vi "Special_Case_Mistake_Resolve-1.vi"(1 "[IN] Subtracks":T1(array[cluster]), 2 "[IN] Index of \nBest Subtrack":i32) -> (0 "[OUT] FALSE For Pre\nventing double save":bool)   [LabVIEW 2013]
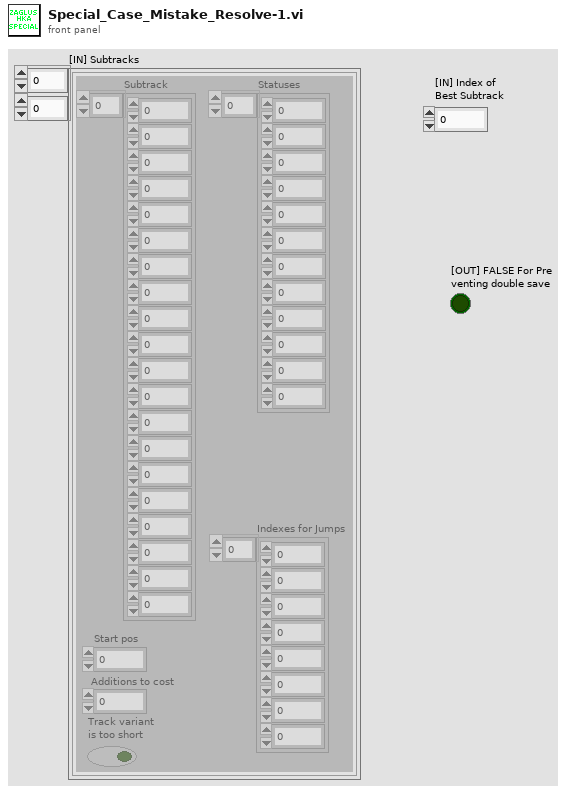
[diagram p1: front panel]
types:
  T1 = cluster{"Subtrack":dbl[], "Statuses":i16[], "Start pos":i32, "Additions to cost":i32, "Track variant \nis too short":bool, "Indexes for Jumps":i32[]}[][]
  T2 = cluster{"Subtrack":dbl[], "Statuses":i16[], "Start pos":i32, "Additions to cost":i32, "Track variant \nis too short":bool, "Indexes for Jumps":i32[]}
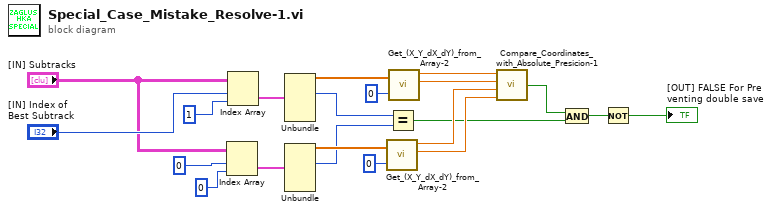
[diagram p0: block diagram]
diagram:
  n1 = Index Array(array="[IN] Subtracks", index (row)=0, index (col)=0 ("index (row)")) -> (element=w16:T2)
  n2 = Index Array(array="[IN] Subtracks", index (row)="[IN] Index of \nBest Subtrack", index (col)=1 ("disabled index (col)")) -> (element=w20:T2)
  n3 = Unbundle(w20) -> ("Subtrack"=w15:dbl[], "Start pos"=w11:i32)  [unwired: 4 out]
  n4 = Unbundle(w16) -> ("Subtrack"=w12:dbl[], "Start pos"=w10:i32)  [unwired: 4 out]
  n5 = call "Get_(X_Y_dX_dY)_from_Array-2.vi"("(X,Y,dX,dY)"=w12, "Index of Displacement"=0) -> ("X"=w7:dbl, "Y"=w6:dbl)  [unwired: 2 out]
  n6 = Equal?(x=w11, y=w10) -> (x = y?=w4:bool)
  n7 = call "Get_(X_Y_dX_dY)_from_Array-2.vi"("(X,Y,dX,dY)"=w15, "Index of Displacement"=0) -> ("X"=w9:dbl, "Y"=w8:dbl)  [unwired: 2 out]
  n8 = call "Compare_Coordinates_with_Absolute_Presicion-1.vi"("X 1"=w9, "Y 1"=w8, "X 2"=w7, "Y 2"=w6) -> ("[OUT] Same coordinates?"=w5:bool)  [unwired: 1 in]
  n9 = And(x=w5, y=w4) -> (x .and. y?=w3:bool)
  n10 = Not(x=w3) -> (.not. x?=→"[OUT] FALSE For Pre\nventing double save":bool)
